vi "MainControlVI.vi"() -> ()   [LabVIEW 2016]
panel:
  in  "STOP":bool
  in  "Raw (V)":dbl
  out "Temperature (C)":dbl format="%#_13g"
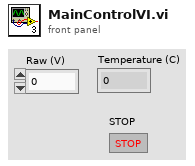
[diagram p1: front panel]
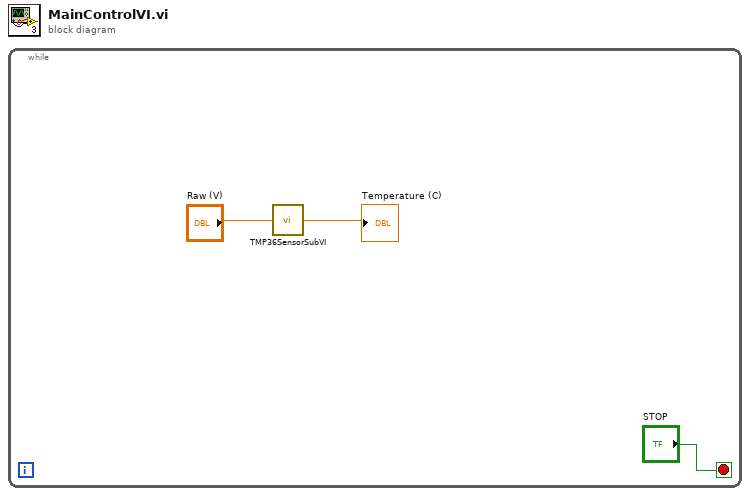
[diagram p0: block diagram]
diagram:
  n1 = while {
    stop <- "STOP" stop-if-true
    n2 = call "TMP36SensorSubVI.vi"("Raw Input (V)"="Raw (V)") -> ("Temperature (C)"=→"Temperature (C)":dbl)
  }
